vi "reportGenMain.vi"(8 "Error In":errorcluster) -> (0 "Error Out":errorcluster)   [LabVIEW 2018]
panel:
  out "Result Table":string[][](table)
  in  "Export Button":bool
  in  "Fetch Button":bool
  in  "To Date":timestamp format="%<%Y/%m/%d %H:%M>T"
  in  "From Date":timestamp format="%<%Y/%m/%d %H:%M>T"
  in  "Stop":bool
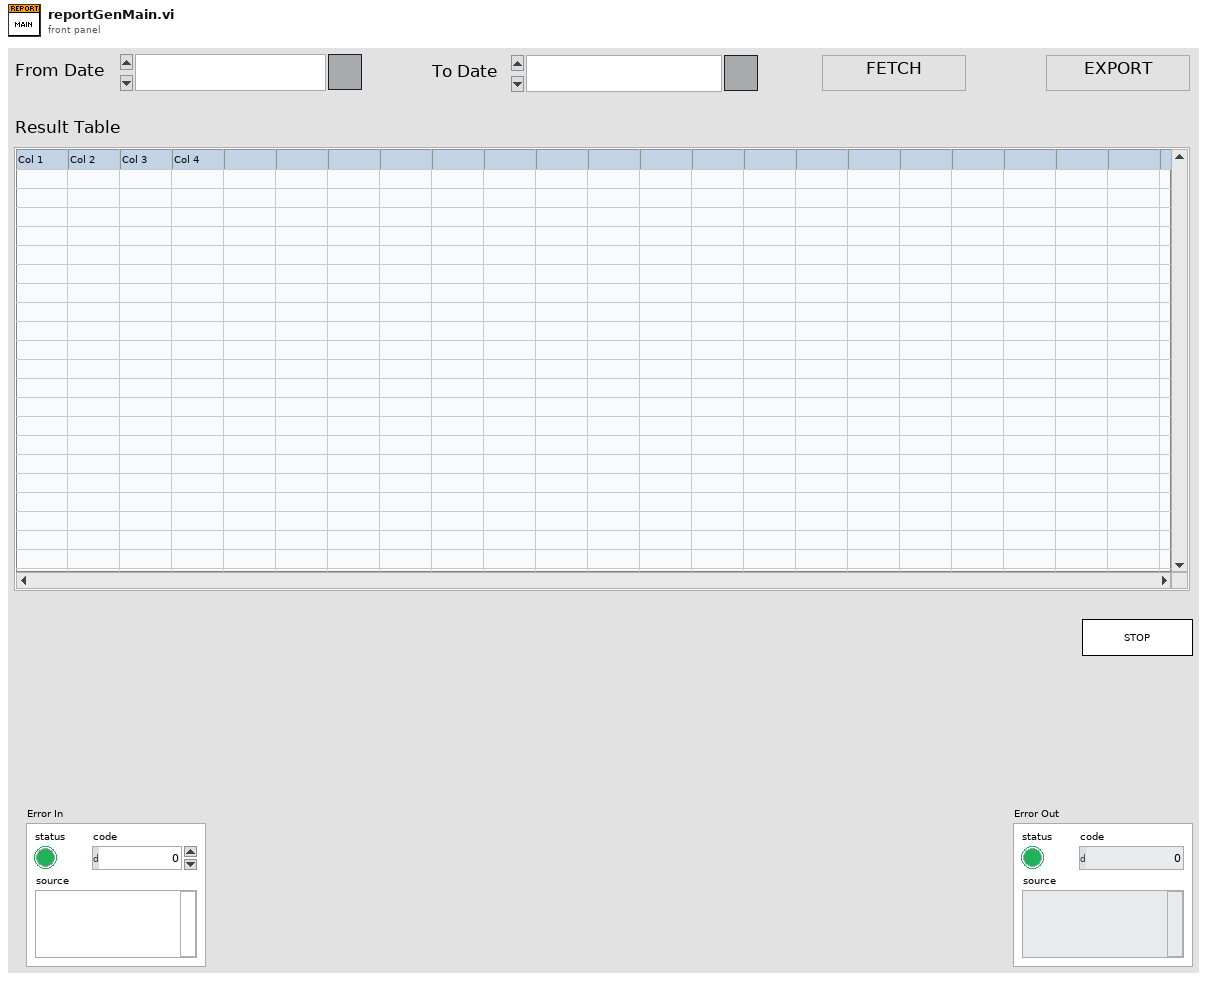
[diagram p1: front panel]
types:
  T1 = enum32{"Invalid", "Standard", "Closed", "Hidden", "Minimized", "Maximized"}
  T2 = enum32{"invalid app kind", "Development System", "Run Time System", "Student Edition", "Embedded LabVIEW", "Evaluation", "Custom"}
  T3 = cluster{"Core":cluster{"Current VI Reference":refnum<vi>, "Close Panel on Exit?":bool}, "From Date":timestamp, "To Date":timestamp, "Result Table":string[][]}
  T4 = cluster{"Current VI Reference":refnum<vi>, "Close Panel on Exit?":bool}
  T5 = typedef "pathCluster.ctl" = cluster{"src Folder Path":path, "Controller Module Path":path, "UI Module Path":path, "Model Select Module Path":path, "Barcode Printer Module Path":path, "Barcode Scanner Module Path":path, "Database Module Path":path, "Report Generation Path":path, "Simulation Path":path, "subVIs Folder Path":path, "info Folder Path":path, "config file Path":path, "cutomerLogo Path":path}
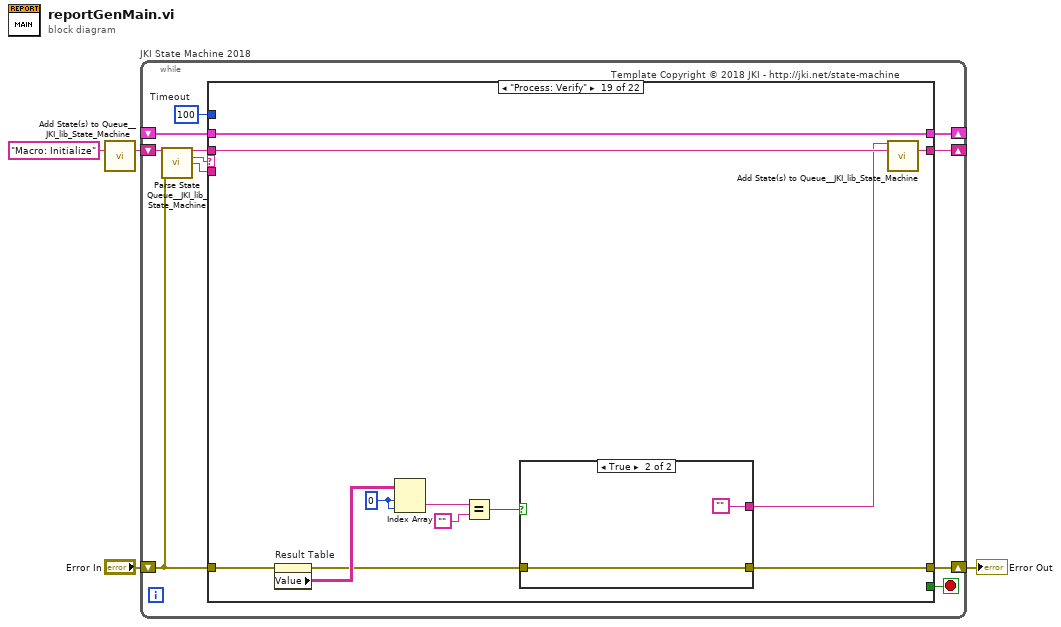
[diagram p0: block diagram]
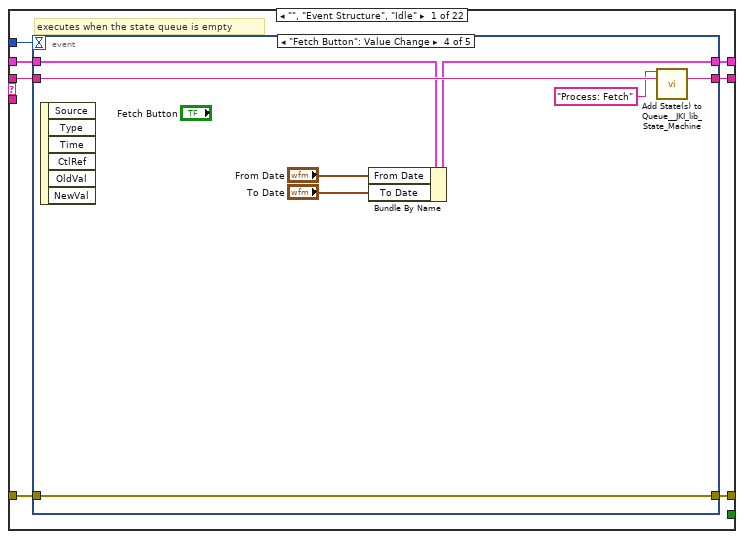
[diagram p2: hidden frame]
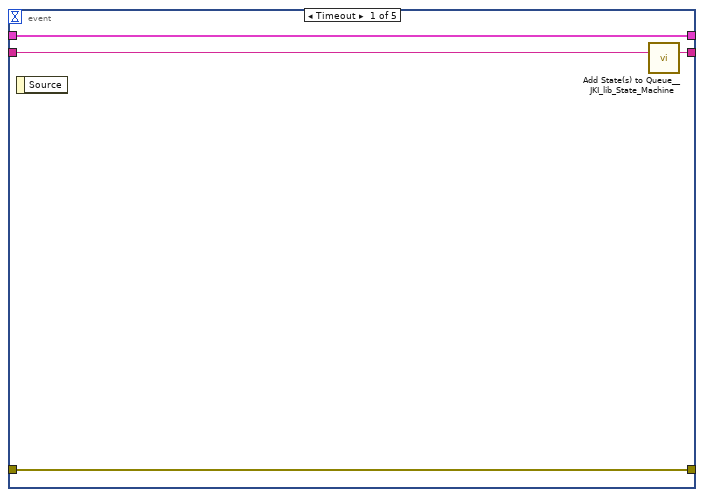
[diagram p3: hidden frame]
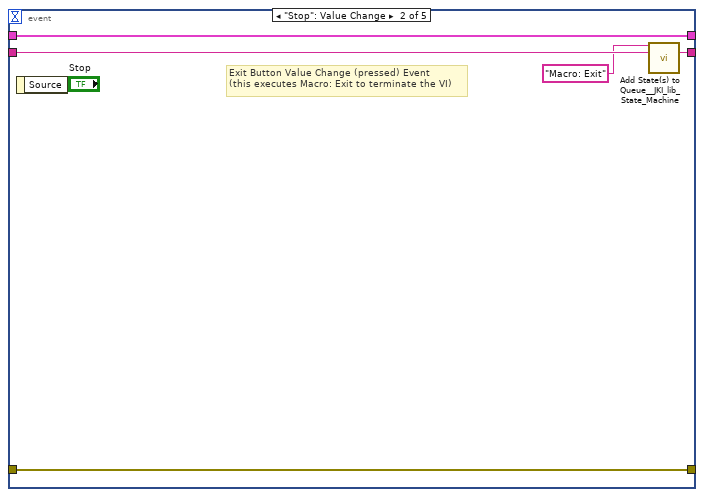
[diagram p4: hidden frame]
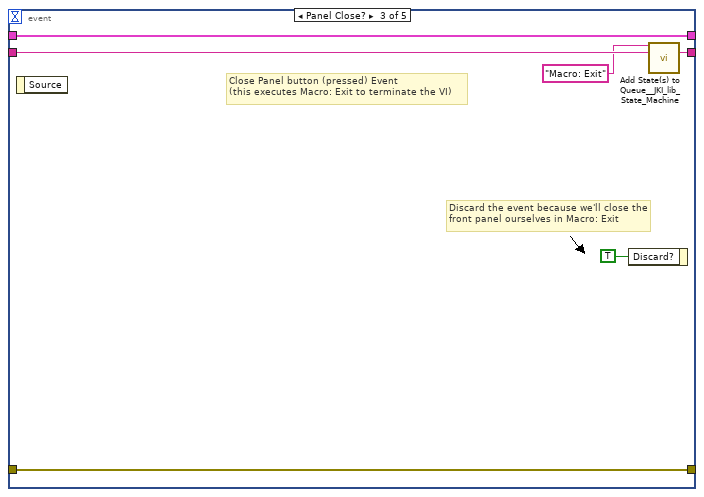
[diagram p5: hidden frame]
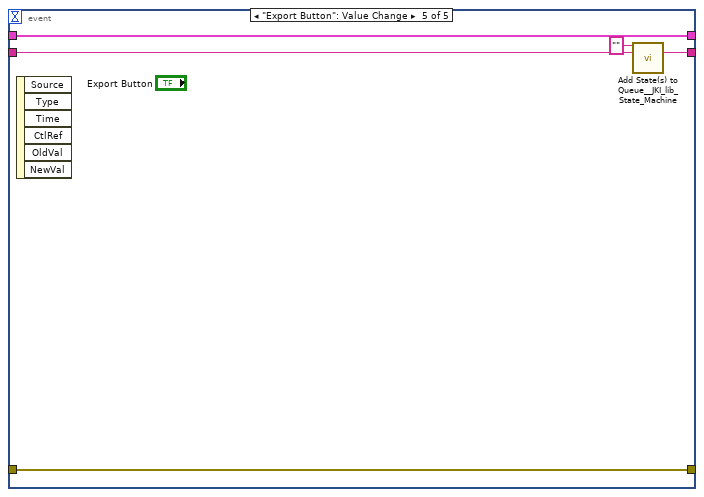
[diagram p6: hidden frame]
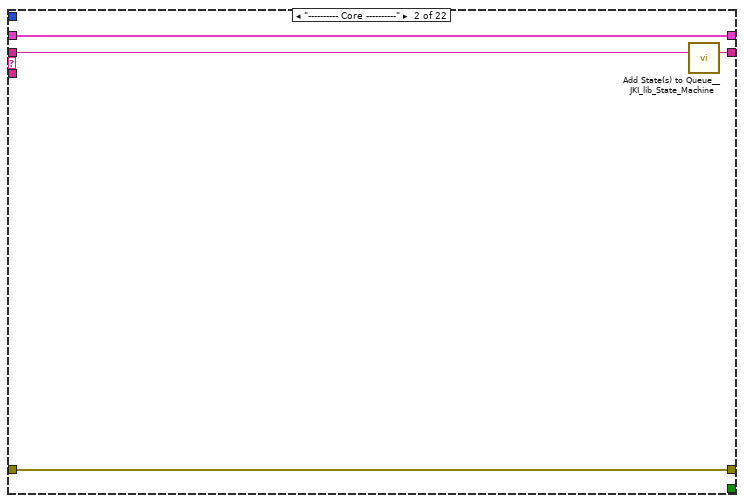
[diagram p7: hidden frame]
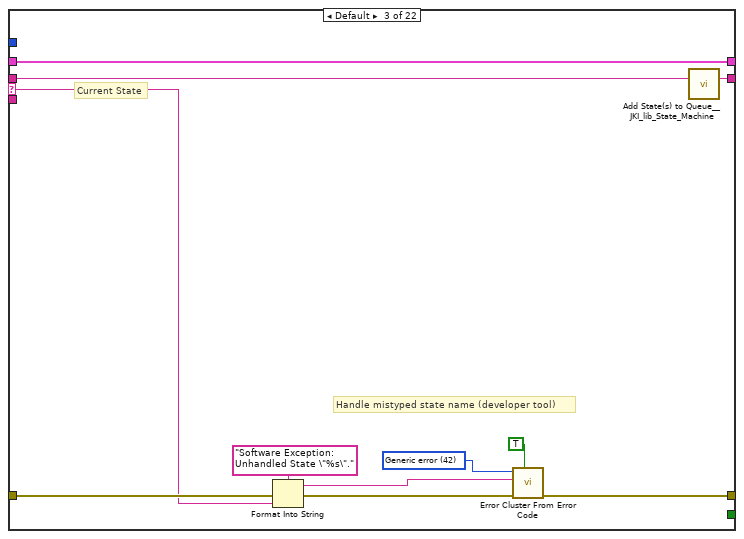
[diagram p8: hidden frame]
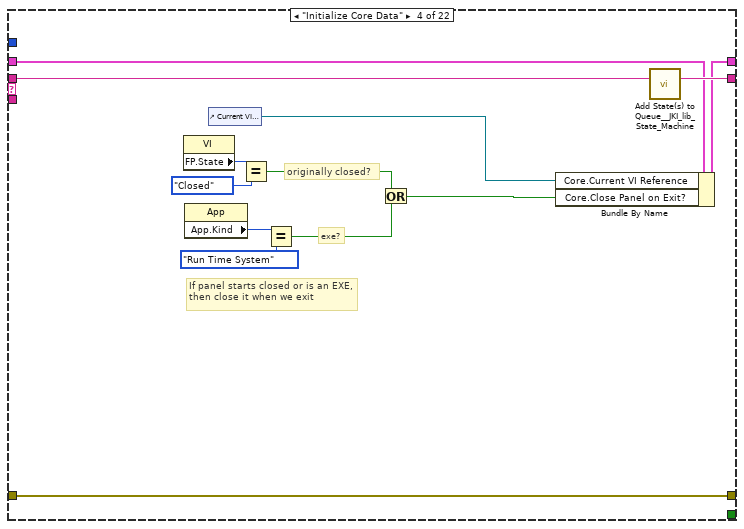
[diagram p9: hidden frame]
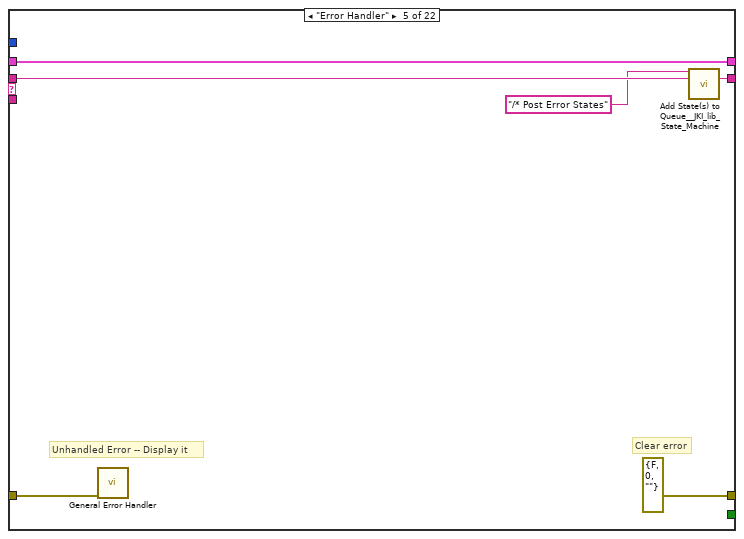
[diagram p10: hidden frame]
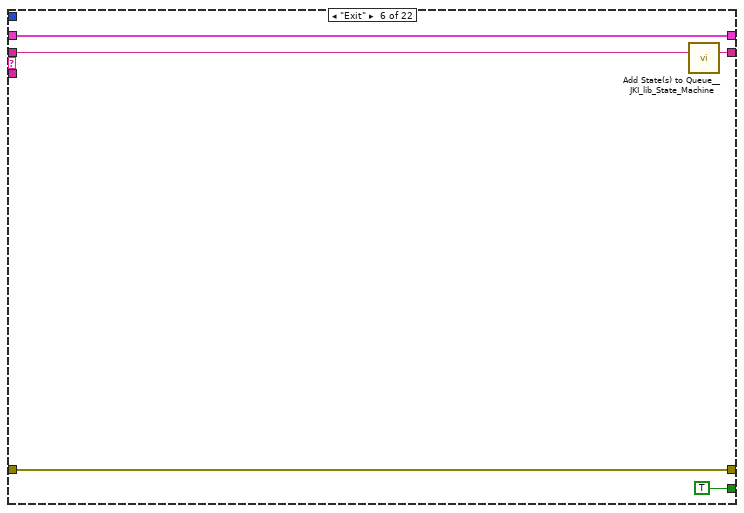
[diagram p11: hidden frame]
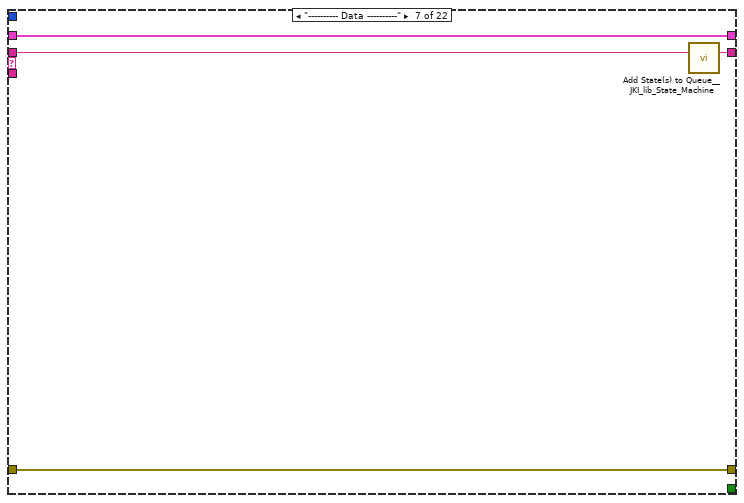
[diagram p12: hidden frame]
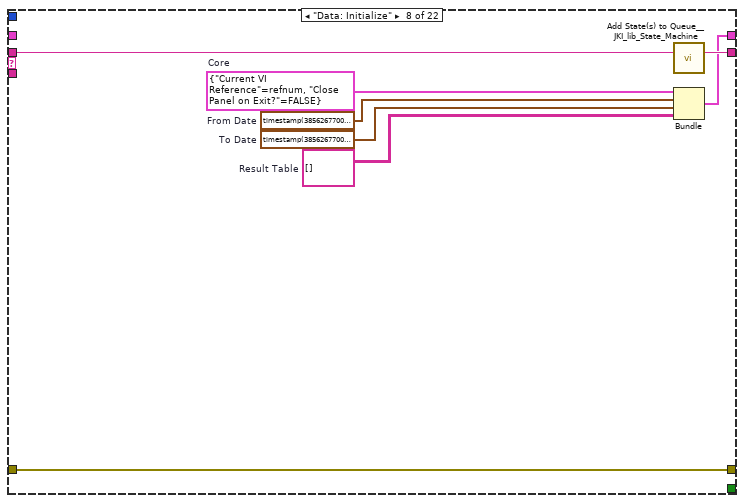
[diagram p13: hidden frame]
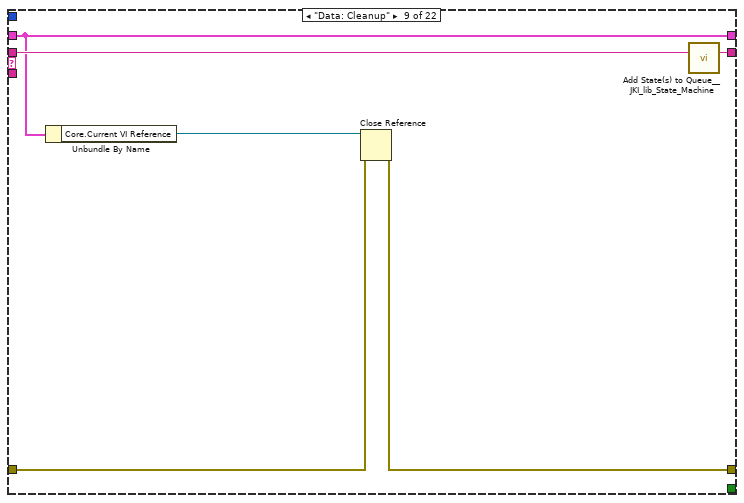
[diagram p14: hidden frame]
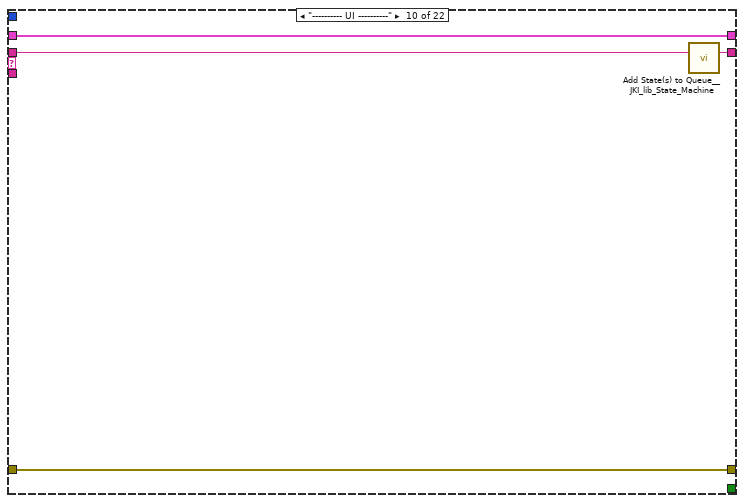
[diagram p15: hidden frame]
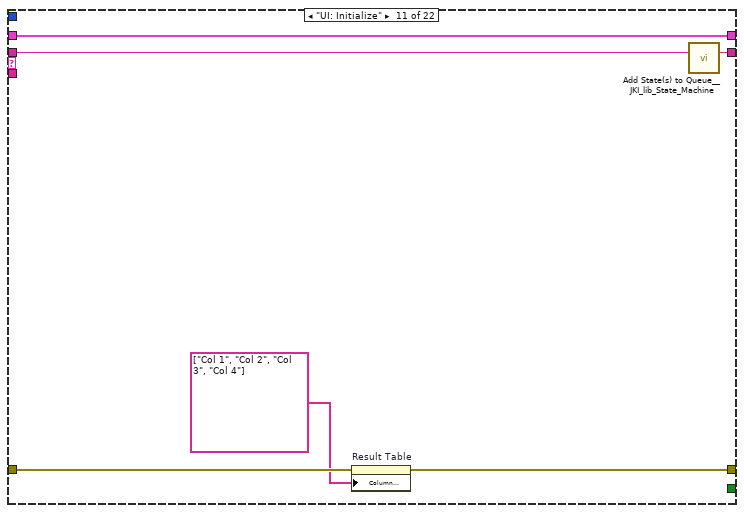
[diagram p16: hidden frame]
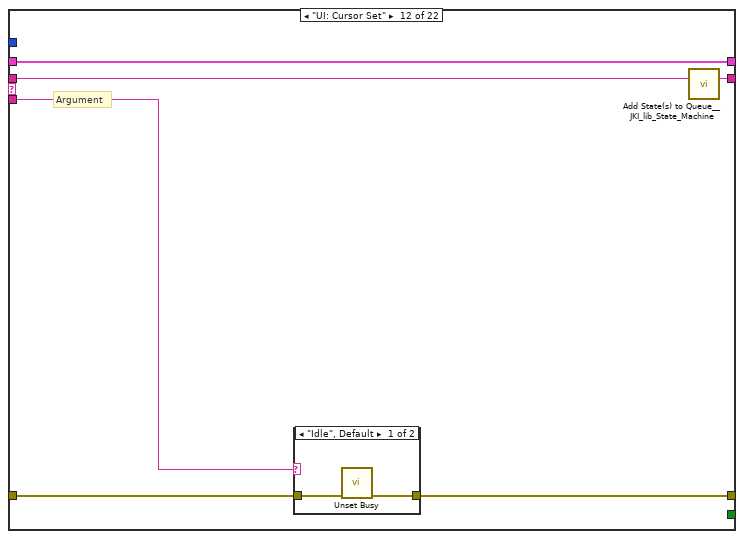
[diagram p17: hidden frame]
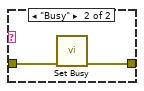
[diagram p18: hidden frame]
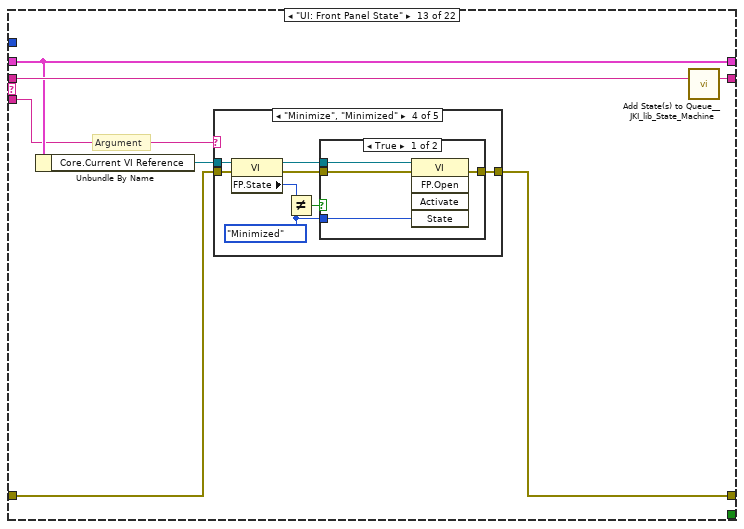
[diagram p19: hidden frame]
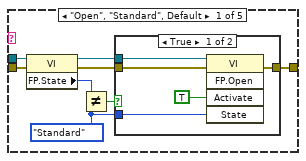
[diagram p20: hidden frame]
diagram:
  n1 = call <vilib>:"Add State(s) to Queue__JKI_lib_State_Machine.vi"("State(s) in (\"\")"="Macro: Initialize") -> ("States Out"=w4:string)  [unwired: 14 in]
  n2 = while "JKI State Machine 2018" {
    shift-right: [w8] -> _
    shift-left: _ -> [w7]
    shift-right: [w11] -> w2
    shift-left: "Error In" -> [w5]
    shift-right: [w10] -> _
    shift-left: w4 -> [w12]
    stop <- w9 stop-if-true
    w6 = 100  # Timeout
    # "Template Copyright © 2018 JKI - http://jki.net/state-machine"
    n3 = call <vilib>:"Parse State Queue__JKI_lib_State_Machine.vi"("State Queue"=w12, "Error In (no error)"=w5) -> ("Remaining States"=w14:string, "Current State"=w15:string, "Arguments"=w13:string)  [unwired: 11 in]
    n4 = case shown="\"Process: Verify\"" w15 {
      selector: w15 -> [_ _ w55 _ _ _ _ _ _ _ _ _ _ _ _ _ _ _ _ _ _ _]
      tunnel: w14 -> [w22 w54 w59 w78 w84 w89 w93 w101 w107 w111 w117 w123 w134 w203 w208 w218 w222 w233 w245 w253 w257 w262]
      tunnel: w13 -> [_ _ _ _ _ _ _ _ _ _ _ w118 w128 _ _ _ _ _ _ _ _ _]
      tunnel: w7 -> [w20 w51 w57 w71 w81 w87 w90 _ w102 w108 w115 w121 w130 w200 w205 w215 w219 w231 w243 w250 w254 w259]
      tunnel: [w19 w52 w61 w75 errorcluster {"status"=FALSE, "code"=0, "source"=""} ("error out") w86 w91 w98 w103 w109 w113 w119 w131 w201 w206 w216 w220 w230 w234 w251 w255 w260] -> w11
      tunnel: w5 -> [w18 w52 w60 w75 w80 w86 w91 w98 w104 w109 w114 w120 w132 w201 w206 w216 w220 w229 w242 w251 w255 w260]
      tunnel: [w21 w53 w58 w77 w83 w88 w92 w100 w106 w110 w116 w122 w133 w202 w207 w217 w221 w232 w244 w252 w256 w261] -> w10
      tunnel: [_ _ _ _ _ TRUE _ _ _ _ _ _ _ _ _ _ _ _ _ _ _ _] -> w9
      tunnel: [w17 w51 w57 w76 w81 w87 w90 w99 w102 w108 w115 w121 w130 w200 w205 w215 w219 w231 w243 w250 w254 w259] -> w8
      tunnel: w6 -> [w16 _ _ _ _ _ _ _ _ _ _ _ _ _ _ _ _ _ _ _ _ _]
      frame "", "Event Structure", "Idle" {
        # "executes when the state queue is empty"
        n5 = event shown="[3] \"Fetch Button\": Value Change" {
          selector: _ -> [_ _ _ _ _]
          dyn-events: _ -> [_ _ _ _ _]
          timeout: w16 -> [_ _ _ _ _]
          tunnel: w22 -> [w26 w31 w37 w44 w48]
          tunnel: [w25 w30 w36 w43 w47] -> w21
          tunnel: w20 -> [w23 w28 w34 w41 w50]
          tunnel: [w24 w29 w35 w45 w49] -> w19
          tunnel: w18 -> [w24 w29 w35 w45 w49]
          tunnel: [w23 w28 w34 w40 w50] -> w17
          event Timeout {
            n6 = event-data() -> ()  [unwired: 1 in, 1 out]
            n7 = call <vilib>:"Add State(s) to Queue__JKI_lib_State_Machine.vi"("State(s) in (\"\")"=w26) -> ("States Out"=w25:string)  [unwired: 14 in]
          }
          event "Stop": Value Change {
            # "Exit Button Value Change (pressed) Event\n(this executes Macro: Exit to terminate the VI)"
            n8 = event-data() -> ()  [unwired: 1 in, 1 out]
            n9 = call <vilib>:"Add State(s) to Queue__JKI_lib_State_Machine.vi"("State(s) in Front (\"\")"="Macro: Exit", "State(s) in (\"\")"=w31) -> ("States Out"=w30:string)  [unwired: 13 in]
          }
          event Panel Close? {
            # "Discard the event because we'll close the front panel ourselves in Macro: Exit"
            # "Close Panel button (pressed) Event\n(this executes Macro: Exit to terminate the VI)"
            n10 = event-data() -> ()  [unwired: 1 in, 1 out]
            n11 = event-data("Discard?"=TRUE) -> ()  [unwired: 1 in, 1 out]
            n12 = call <vilib>:"Add State(s) to Queue__JKI_lib_State_Machine.vi"("State(s) in Front (\"\")"="Macro: Exit", "State(s) in (\"\")"=w37) -> ("States Out"=w36:string)  [unwired: 13 in]
          }
          event "Fetch Button": Value Change {
            n13 = event-data() -> ()  [unwired: 1 in, 6 out]
            n14 = Bundle By Name(cluster=w41, "From Date"="From Date", "To Date"="To Date") -> (w40:T3)
            n15 = call <vilib>:"Add State(s) to Queue__JKI_lib_State_Machine.vi"("State(s) in Front (\"\")"="Process: Fetch" ("State(s) in Front (\"\")"), "State(s) in (\"\")"=w44) -> ("States Out"=w43:string)  [unwired: 13 in]
          }
          event "Export Button": Value Change {
            n16 = event-data() -> ()  [unwired: 1 in, 6 out]
            n17 = call <vilib>:"Add State(s) to Queue__JKI_lib_State_Machine.vi"("State(s) in Front (\"\")"="" ("State(s) in Front (\"\")"), "State(s) in (\"\")"=w48) -> ("States Out"=w47:string)  [unwired: 13 in]
          }
        }
      }
      frame "---------- Core ----------" {
        n18 = call <vilib>:"Add State(s) to Queue__JKI_lib_State_Machine.vi"("State(s) in (\"\")"=w54) -> ("States Out"=w53:string)  [unwired: 14 in]
      }
      frame Default {
        w64 = 42 items=["No error", "Argument error", "Memory is full", "Out of zone", "End of file", "File already open", "Generic file I/O error", "File not found", "File permission error", "Disk is full", "Duplicate path", "Too many files open", "System feature not enabled", "Resource file not found", "Cannot add resource", "Resource not found", "Image not found", "Image memory error", "Pen does not exist", "Config type invalid", "Config token not found", "Config parse error", "Config memory error", "Bad external code format", "Bad external code offset", "External code not present", "Null window", "Destroy window error", "Null menu", "Print aborted", "Bad print record", "Print driver error", "Windows error during printing", "Memory error during printing", "Print dialog error", "Generic print error", "Invalid device refnum", "Device not found", "Device parameter error", "Device unit error", "Cannot open device", "Device call aborted", "Generic error", "Cancelled by user", "Object ID too low", "Object ID too high", "Object not in heap", "Unknown heap", "Unknown object (invalid DefProc)", "Unknown object (DefProc not in table)", "Message out of range", "Invalid (null) method", "Unknown message", "Manager call not supported", "Bad address", "Network operation in progress", "Network operation timed out", "Connection is busy", "Network attribute not supported", "Network error", "Address in use", "System out of memory", "Connection aborted", "Connection refused", "Not connected", "Already connected", "Connection closed", "Initialization error (interapplication manager)", "Bad occurrence", "Wait on unbound occurrence handler", "Occurrence queue overflow", "Datalog type conflict", "Unused", "Unrecognized type (interapplication manager)", "Memory corrupt", "Failed to make temporary DLL", "Old CIN version", "Drag socket not found", "Failed to load drop-object", "Failed to register OLE object", "Failed to release OLE object", "Format specifier type mismatch", "Unknown format specifier", "Too few format specifiers", "Too many format specifiers", "Scan failed", "Newer CIN version", "Error converting to variant", "Runtime menu error", "Password tampered", "Variant attribute not found", "Incompatible variant data type", "Event data is not available", "Event Store is not present", "Occurrence is not found", "Event Queue is not created", "Event info is not available", "Refnum passed is NULL", "Error retrieving Class GUID", "Error retrieving CoClass GUID", "Error retrieving TypeLib GUID.", "Bad built application magic bytes.", "Specific driver is different from the specific driver associated with the Logical Name.", "There is no session opened to the class driver.", "Max Error", "MAX - Error with config objects", "MAX - Error loading configuration", "MAX - Group not supported"]
        # "Current State"
        # "Handle mistyped state name (developer tool)"
        n19 = Format Into String(format string="Software Exception: Unhandled State \"%s\"." ("message"), error in=w60, w55) -> (resulting string=w63:string, error out=w62:errorcluster)  [unwired: 1 in]
        n20 = call <vilib>:"Error Cluster From Error Code.vi"("show call chain? (False)"=TRUE, "error in (no error)"=w62, "error message (\"\")"=w63, "error code (0)"=w64) -> ("error out"=w61:errorcluster)  [unwired: 5 in]
        n21 = call <vilib>:"Add State(s) to Queue__JKI_lib_State_Machine.vi"("State(s) in (\"\")"=w59) -> ("States Out"=w58:string)  [unwired: 14 in]
      }
      frame "Initialize Core Data" {
        # "originally closed?"
        # "exe?"
        # "If panel starts closed or is an EXE, then close it when we exit"
        n22 = property class="VI"() -> ("FP.State"=w68:T1)  [unwired: 2 in, 2 out]
        n23 = property class="App"() -> ("App.Kind"=w74:T2)  [unwired: 2 in, 2 out]
        n24 = control-ref of="Current VI Reference"() -> (w69:refnum<vi>)
        n25 = Equal?(x=w68, y=T1."Closed" ("Front Panel Window:State")) -> (x = y?=w66:bool)
        n26 = Equal?(x=w74, y=T2."Run Time System" ("Application:Kind")) -> (x = y?=w72:bool)
        n27 = Or(x=w66, y=w72) -> (x .or. y?=w70:bool)
        n28 = Bundle By Name(cluster=w71, "Core.Current VI Reference"=w69, "Core.Close Panel on Exit?"=w70) -> (w76:T3)
        n29 = call <vilib>:"Add State(s) to Queue__JKI_lib_State_Machine.vi"("State(s) in (\"\")"=w78) -> ("States Out"=w77:string)  [unwired: 14 in]
      }
      frame "Error Handler" {
        # "Unhandled Error -- Display it"
        # "Clear error"
        n30 = call <vilib>:"General Error Handler.vi"("error in (no error)"=w80) -> ()  [unwired: 10 in, 5 out]
        n31 = call <vilib>:"Add State(s) to Queue__JKI_lib_State_Machine.vi"("State(s) in Front (\"\")"="/* Post Error States", "State(s) in (\"\")"=w84) -> ("States Out"=w83:string)  [unwired: 13 in]
      }
      frame "Exit" {
        n32 = call <vilib>:"Add State(s) to Queue__JKI_lib_State_Machine.vi"("State(s) in (\"\")"=w89) -> ("States Out"=w88:string)  [unwired: 14 in]
      }
      frame "---------- Data ----------" {
        n33 = call <vilib>:"Add State(s) to Queue__JKI_lib_State_Machine.vi"("State(s) in (\"\")"=w93) -> ("States Out"=w92:string)  [unwired: 14 in]
      }
      frame "Data: Initialize" {
        w94 = string[][] []  # Result Table
        w95 = timestamp(3856267700.8588862 s since 1904-01-01)  # To Date
        w96 = timestamp(3856267700.8588862 s since 1904-01-01)  # From Date
        w97 = T4 {"Current VI Reference"=refnum, "Close Panel on Exit?"=FALSE}  # Core
        n34 = call <vilib>:"Add State(s) to Queue__JKI_lib_State_Machine.vi"("State(s) in (\"\")"=w101) -> ("States Out"=w100:string)  [unwired: 14 in]
        n35 = Bundle("Core"=w97, "From Date"=w96, "To Date"=w95, "Result Table"=w94) -> (w99:T3)  [unwired: 1 in]
      }
      frame "Data: Cleanup" {
        n36 = Unbundle By Name(w102) -> ("Core.Current VI Reference"=w105:refnum<vi>)
        n37 = Close Reference(reference=w105, error in (no error)=w104) -> (error out=w103:errorcluster)
        n38 = call <vilib>:"Add State(s) to Queue__JKI_lib_State_Machine.vi"("State(s) in (\"\")"=w107) -> ("States Out"=w106:string)  [unwired: 14 in]
      }
      frame "---------- UI ----------" {
        n39 = call <vilib>:"Add State(s) to Queue__JKI_lib_State_Machine.vi"("State(s) in (\"\")"=w111) -> ("States Out"=w110:string)  [unwired: 14 in]
      }
      frame "UI: Initialize" {
        n40 = property on="Result Table" class="Tbl (strict)"(error in=w114, "Column Headers[]"=string[] ["Col 1", "Col 2", "Col 3", "Col 4"] ("Column Header Strings[]")) -> (error out=w113:errorcluster)  [unwired: 1 in, 1 out]
        n41 = call <vilib>:"Add State(s) to Queue__JKI_lib_State_Machine.vi"("State(s) in (\"\")"=w117) -> ("States Out"=w116:string)  [unwired: 14 in]
      }
      frame "UI: Cursor Set" {
        # "Argument"
        n42 = case shown="\"Idle\", Default" w118 {
          tunnel: w120 -> [w125 w127]
          tunnel: [w124 w126] -> w119
          frame "Idle", Default {
            n43 = call <vilib>:"Unset Busy.vi"("error in (no error)"=w125) -> ("error out"=w124:errorcluster)  [unwired: 10 in]
          }
          frame "Busy" {
            n44 = call <vilib>:"Set Busy.vi"("error in (no error)"=w127) -> ("error out"=w126:errorcluster)  [unwired: 9 in, 1 out]
          }
        }
        n45 = call <vilib>:"Add State(s) to Queue__JKI_lib_State_Machine.vi"("State(s) in (\"\")"=w123) -> ("States Out"=w122:string)  [unwired: 14 in]
      }
      frame "UI: Front Panel State" {
        # "Argument"
        n46 = Unbundle By Name(w130) -> ("Core.Current VI Reference"=w129:refnum<vi>)
        n47 = case shown="\"Minimize\", \"Minimized\"" w128 {
          tunnel: w132 -> [w140 w155 w166 w179 w192]
          tunnel: [w142 w156 w168 w181 w194] -> w131
          tunnel: w129 -> [w141 w153 w167 w180 w193]
          frame "Open", "Standard", Default {
            w135 = T1."Standard" ("State")
            n48 = property class="VI"(reference=w141, error in=w140) -> (reference out=w138:refnum<vi>, error out=w139:errorcluster, "FP.State"=w137:T1)
            n49 = Not Equal?(x=w137, y=w135) -> (x != y?=w136:bool)
            n50 = case shown="True" w136 {
              tunnel: [w146 w148] -> w142
              tunnel: w139 -> [w145 w148]
              tunnel: w138 -> [w144 _]
              tunnel: w135 -> [w143 _]
              frame True {
                n51 = invoke class="VI" method="FP.Open"(reference=w144, error in=w145, "Activate"=TRUE, "State"=w143) -> (error out=w146:errorcluster)  [unwired: 1 in, 4 out]
              }
              frame False {
              }
            }
          }
          frame "Close", "Closed" {
            n52 = property class="VI"(reference=w153, error in=w155) -> (reference out=w152:refnum<vi>, error out=w154:errorcluster, "FP.State"=w150:T1)
            n53 = Not Equal?(x=w150, y=T1."Closed" ("Front Panel Window:State")) -> (x != y?=w149:bool)
            n54 = case shown="True" w149 {
              tunnel: [w157 w160] -> w156
              tunnel: w154 -> [w157 w159]
              tunnel: w152 -> [_ w158]
              frame False {
              }
              frame True {
                n55 = invoke class="VI" method="FP.Close"(reference=w158, error in=w159) -> (error out=w160:errorcluster)  [unwired: 1 in, 2 out]
              }
            }
          }
          frame "Hidden", "Hide" {
            w161 = T1."Hidden" ("State")
            n56 = property class="VI"(reference=w167, error in=w166) -> (reference out=w164:refnum<vi>, error out=w165:errorcluster, "FP.State"=w163:T1)
            n57 = Not Equal?(x=w163, y=w161) -> (x != y?=w162:bool)
            n58 = case shown="True" w162 {
              tunnel: [w172 w173] -> w168
              tunnel: w165 -> [w171 w173]
              tunnel: w164 -> [w170 _]
              tunnel: w161 -> [w169 _]
              frame True {
                n59 = invoke class="VI" method="FP.Open"(reference=w170, error in=w171, "State"=w169) -> (error out=w172:errorcluster)  [unwired: 2 in, 4 out]
              }
              frame False {
              }
            }
          }
          frame "Minimize", "Minimized" {
            w174 = T1."Minimized" ("State")
            n60 = property class="VI"(reference=w180, error in=w179) -> (reference out=w177:refnum<vi>, error out=w178:errorcluster, "FP.State"=w176:T1)
            n61 = Not Equal?(x=w176, y=w174) -> (x != y?=w175:bool)
            n62 = case shown="True" w175 {
              tunnel: [w185 w186] -> w181
              tunnel: w178 -> [w184 w186]
              tunnel: w177 -> [w183 _]
              tunnel: w174 -> [w182 _]
              frame True {
                n63 = invoke class="VI" method="FP.Open"(reference=w183, error in=w184, "State"=w182) -> (error out=w185:errorcluster)  [unwired: 2 in, 4 out]
              }
              frame False {
              }
            }
          }
          frame "Maximize", "Maximized" {
            w187 = T1."Maximized" ("State")
            n64 = property class="VI"(reference=w193, error in=w192) -> (reference out=w190:refnum<vi>, error out=w191:errorcluster, "FP.State"=w189:T1)
            n65 = Not Equal?(x=w189, y=w187) -> (x != y?=w188:bool)
            n66 = case shown="True" w188 {
              tunnel: [w198 w199] -> w194
              tunnel: w191 -> [w197 w199]
              tunnel: w190 -> [w196 _]
              tunnel: w187 -> [w195 _]
              frame True {
                n67 = invoke class="VI" method="FP.Open"(reference=w196, error in=w197, "State"=w195) -> (error out=w198:errorcluster)  [unwired: 2 in, 4 out]
              }
              frame False {
              }
            }
          }
        }
        n68 = call <vilib>:"Add State(s) to Queue__JKI_lib_State_Machine.vi"("State(s) in (\"\")"=w134) -> ("States Out"=w133:string)  [unwired: 14 in]
      }
      frame "---------- Macro ----------" {
        n69 = call <vilib>:"Add State(s) to Queue__JKI_lib_State_Machine.vi"("State(s) in (\"\")"=w203) -> ("States Out"=w202:string)  [unwired: 14 in]
      }
      frame "Macro: Initialize" {
        w204 = "Data: Initialize\nInitialize Core Data\nUI: Initialize\nUI: Front Panel State >> Open"  # Data: Initialize Initialize Core Data UI: Initialize UI: Front Panel State >> Open
        n70 = call <vilib>:"Add State(s) to Queue__JKI_lib_State_Machine.vi"("State(s) in Front (\"\")"=w204, "State(s) in (\"\")"=w208) -> ("States Out"=w207:string)  [unwired: 13 in]
      }
      frame "Macro: Exit" {
        n71 = Unbundle By Name(w215) -> ("Core.Close Panel on Exit?"=w214:bool)
        n72 = Select(t="UI: Front Panel State >> Close", s=w214, f="") -> (s? t:f=w211:string)
        n73 = call <vilib>:"Add State(s) to Queue__JKI_lib_State_Machine.vi"("State(s) in (\"\")"=w211, "State(s) at Back (\"\")"="Data: Cleanup\nExit") -> ("States Out"=w209:string)  [unwired: 13 in]
        n74 = call <vilib>:"Add State(s) to Queue__JKI_lib_State_Machine.vi"("State(s) in Front (\"\")"=w209, "State(s) in (\"\")"=w218) -> ("States Out"=w217:string)  [unwired: 13 in]
      }
      frame "---------- Process ----------" {
        n75 = call <vilib>:"Add State(s) to Queue__JKI_lib_State_Machine.vi"("State(s) in (\"\")"=w222) -> ("States Out"=w221:string)  [unwired: 14 in]
      }
      frame "Process: Fetch" {
        n76 = call "getPaths.vi"("Error In"=w229) -> ("Error Out"=w228:errorcluster, "Application Path Cluster"=w227:T5)  [unwired: 9 in]
        n77 = Unbundle By Name(w227) -> ("info Folder Path"=w226:path)
        n78 = Build Path(base path=w226, name or relative path="database.udl") -> (appended path=w224:path)
        n79 = call "queryAndFetch.vi"("Error In"=w228, "Query"="", "DB File Path"=w224) -> ("Error Out"=w230:errorcluster)  [unwired: 7 in, 1 out]
        n80 = call <vilib>:"Add State(s) to Queue__JKI_lib_State_Machine.vi"("State(s) in (\"\")"=w233) -> ("States Out"=w232:string)  [unwired: 14 in]
      }
      frame "Process: Verify" {
        w240 = 0 ("index (row)")
        n81 = property on="Result Table" class="Tbl (strict)"(error in=w242) -> (error out=w235:errorcluster, "Value"=w241:string[][])  [unwired: 1 in, 1 out]
        n82 = Index Array(array=w241, index (row)=w240, index (col)=w240) -> (element=w239:string)
        n83 = Equal?(x=w239, y="") -> (x = y?=w237:bool)
        n84 = case shown="True" w237 {
          tunnel: ["Process: Export" ""] -> w236
          tunnel: w235 -> [w246 w248]
          tunnel: [w246 w248] -> w234
          frame False {
          }
          frame True {
          }
        }
        n85 = call <vilib>:"Add State(s) to Queue__JKI_lib_State_Machine.vi"("State(s) in Front (\"\")"=w236, "State(s) in (\"\")"=w245) -> ("States Out"=w244:string)  [unwired: 13 in]
      }
      frame "Process: Export" {
        n86 = call <vilib>:"Add State(s) to Queue__JKI_lib_State_Machine.vi"("State(s) in (\"\")"=w253) -> ("States Out"=w252:string)  [unwired: 14 in]
      }
      frame "---------- Display ----------" {
        n87 = call <vilib>:"Add State(s) to Queue__JKI_lib_State_Machine.vi"("State(s) in (\"\")"=w257) -> ("States Out"=w256:string)  [unwired: 14 in]
      }
      frame "Display: Result" {
        n88 = Unbundle By Name(w259) -> ("Result Table"=→"Result Table":string[][])
        n89 = call <vilib>:"Add State(s) to Queue__JKI_lib_State_Machine.vi"("State(s) in (\"\")"=w262) -> ("States Out"=w261:string)  [unwired: 14 in]
      }
    }
  }
  "Error Out" <- w2
